vi "f1.vi"(1 "Numeric":dbl) -> (0 "Numeric 2":dbl)   [LabVIEW 2020]
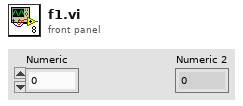
[diagram p1: front panel]
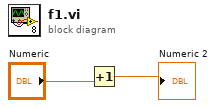
[diagram p0: block diagram]
diagram:
  n1 = Increment(x="Numeric") -> (x+1=→"Numeric 2":dbl)
